vi "Tab Control Ref.vi"(4 "Control Names to exlude":string[](array[string])=["error in (no error)", "error out", "Debug Abort"], 6 "Control State(Enable)":T1(ring), 8 "error in":errorcluster, 11 "TabControl Reference":refnum<vi>) -> (0 "error out":errorcluster)   [LabVIEW 2018]
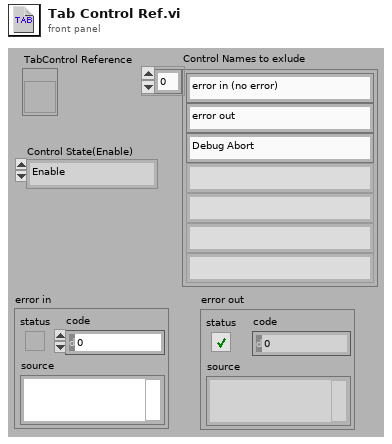
[diagram p1: front panel]
types:
  T1 = enum8{"Enable", "Disabled", "Disabled and Grayed"}
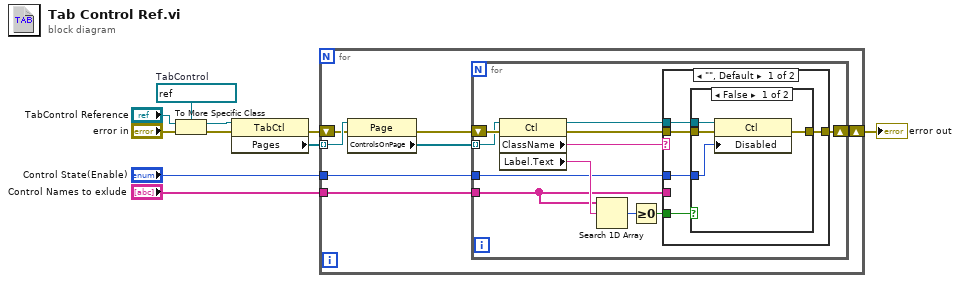
[diagram p0: block diagram]
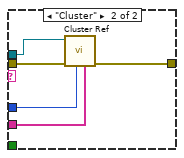
[diagram p3: hidden frame]
diagram:
  w8 = refnum<vi> refnum  # TabControl
  n1 = To More Specific Class(target class=w8, reference="TabControl Reference", error in="error in") -> (specific class reference=w6:refnum<vi>, error out=w4:errorcluster)
  n2 = property class="TabCtl"(reference=w6, error in=w4) -> (error out=w10:errorcluster, "Pages"=w9:refnum<vi>[])  [unwired: 1 out]
  n3 = for {
    tunnel: w9 -> [w17] mode=indexing
    tunnel: "Control Names to exlude" -> [w13]
    tunnel: "Control State(Enable)" -> [w12]
    shift-right: [w11] -> w1
    shift-left: w10 -> [w15]
    n4 = property class="Page"(reference=w17, error in=w15) -> (error out=w14:errorcluster, "ControlsOnPage"=w16:refnum<vi>[])  [unwired: 1 out]
    n5 = for {
      tunnel: w16 -> [w19] mode=indexing
      tunnel: w13 -> [w18]
      tunnel: w12 -> [w21]
      shift-right: [w20] -> w11
      shift-left: w14 -> [w28]
      n6 = property class="Ctl"(reference=w19, error in=w28) -> (reference out=w26:refnum<vi>, error out=w25:errorcluster, "ClassName"=w27:string, "Label.Text"=w22:string)
      n7 = Search 1D Array(1D array=w18, element=w22) -> (index of element=w24:i32)  [unwired: 1 out]
      n8 = Greater Or Equal To 0?(x=w24) -> (x >= 0?=w23:bool)
      n9 = case shown="\"\", Default" w27 {
        tunnel: w26 -> [w29 w41]
        tunnel: w25 -> [w31 w43]
        tunnel: w23 -> [w33 _]
        tunnel: w21 -> [w32 w40]
        tunnel: [w30 w42] -> w20
        tunnel: w18 -> [_ w39]
        frame "", Default {
          n10 = case shown="False" w33 {
            tunnel: w32 -> [w37 _]
            tunnel: w31 -> [w36 w38]
            tunnel: [w35 w38] -> w30
            tunnel: w29 -> [w34 _]
            frame False {
              n11 = property class="Ctl"(reference=w34, error in=w36, "Disabled"=w37) -> (error out=w35:errorcluster)  [unwired: 1 out]
            }
            frame True {
            }
          }
        }
        frame "Cluster" {
          n12 = call "Cluster Ref.vi"("Control Names to exlude"=w39, "Control State(Enable)"=w40, "error in"=w43, "Cluster Reference"=w41) -> ("error out"=w42:errorcluster)  [unwired: 7 in]
        }
      }
    }
  }
  "error out" <- w1
